vi "TCP-Main.vi"() -> ()   [LabVIEW 2014]
panel:
  out "读":string
  in  "Send":bool
  out "错误输出":errorcluster
  in  "错误输入（无错误）":errorcluster
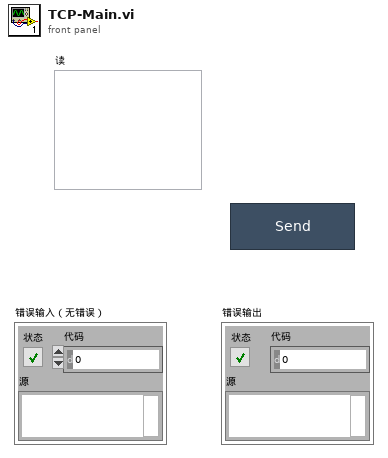
[diagram p1: front panel]
types:
  T1 = enum16{"Init", "Loop", "Write LOFF", "Write LON", "Read", "Exit", "Open", "Close"}
  T2 = enum16{"Standard", "Buffered", "CRLF", "Immediate"}
  T3 = enum32{"invalid app kind", "Development System", "Run Time System", "Student Edition", "Embedded LabVIEW", "Evaluation", "Custom"}
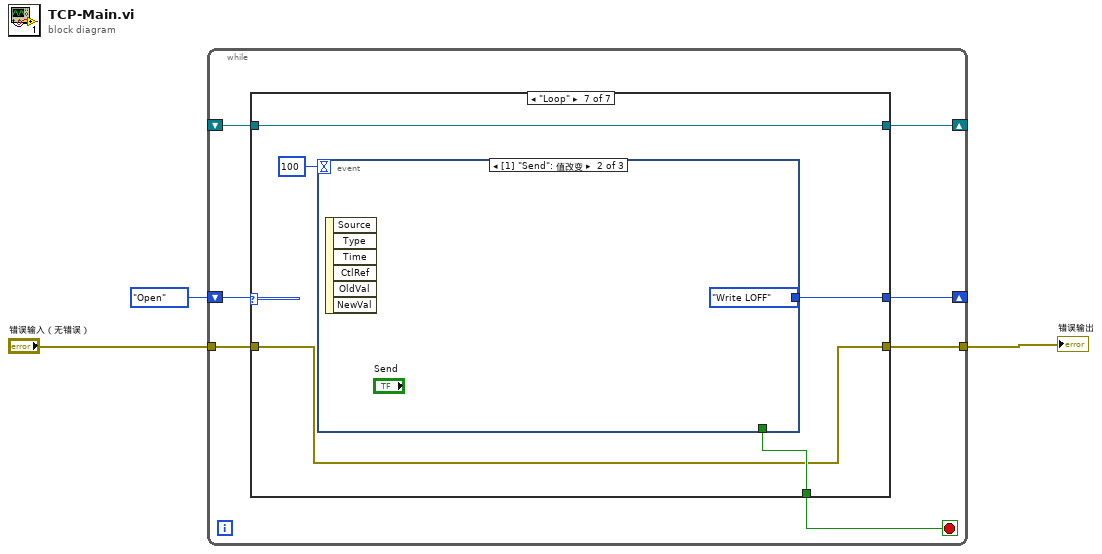
[diagram p0: block diagram]
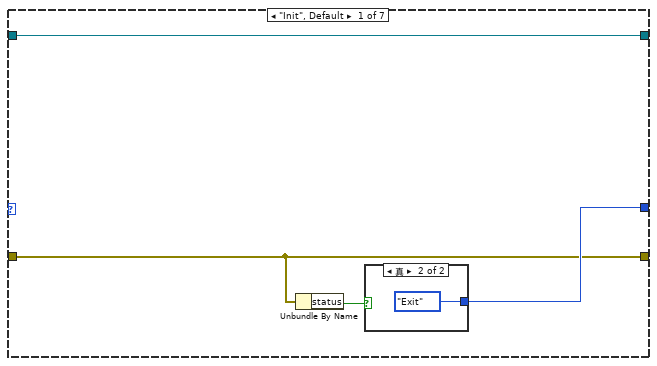
[diagram p2: hidden frame]
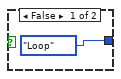
[diagram p3: hidden frame]
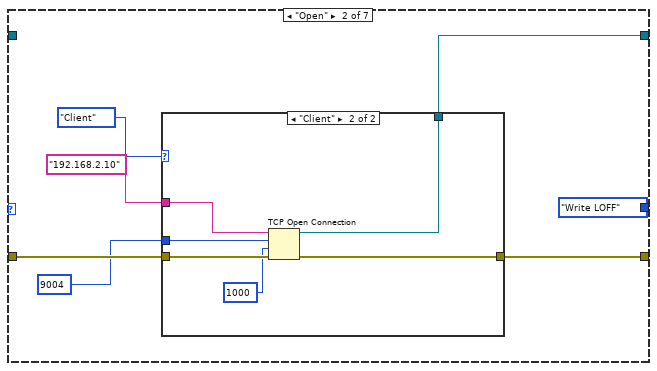
[diagram p4: hidden frame]
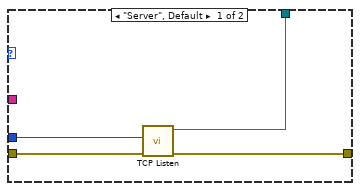
[diagram p5: hidden frame]
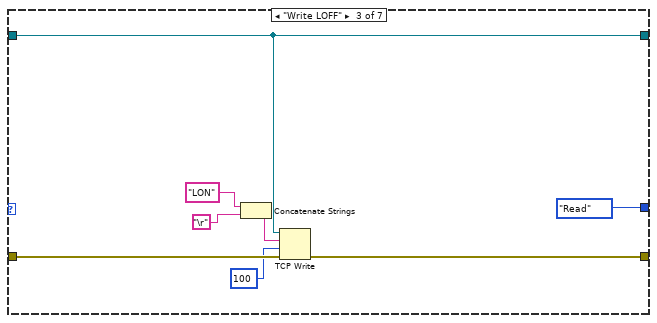
[diagram p6: hidden frame]
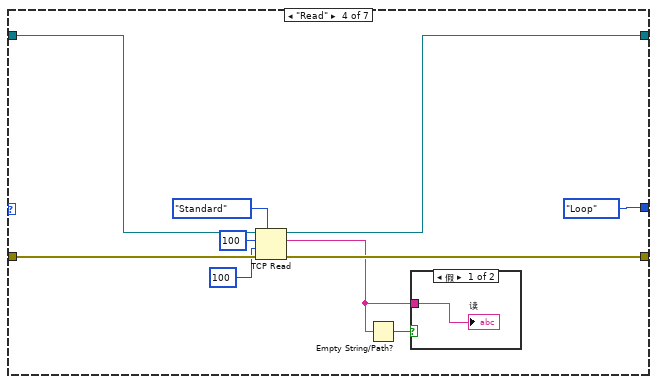
[diagram p7: hidden frame]
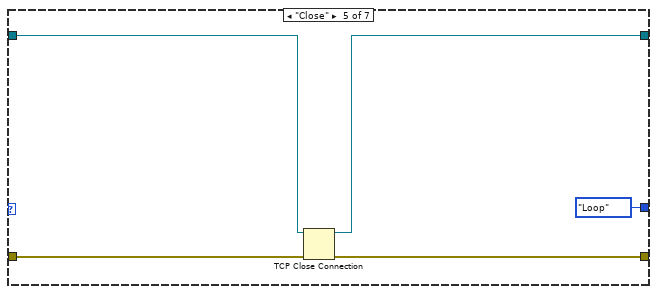
[diagram p9: hidden frame]
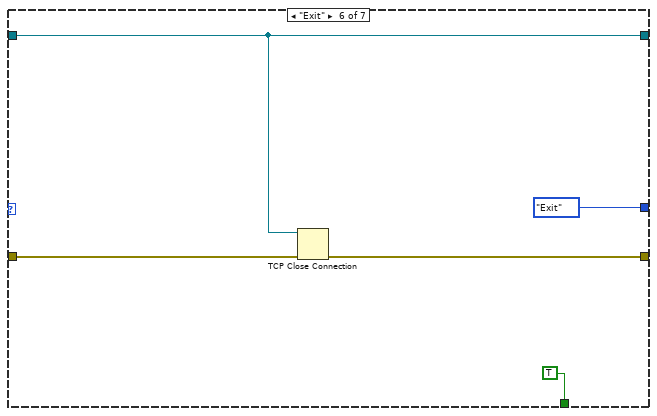
[diagram p10: hidden frame]
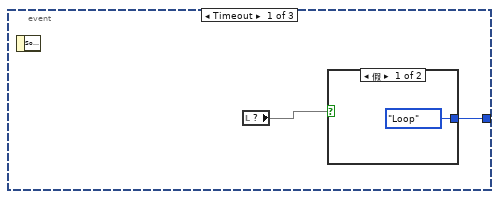
[diagram p11: hidden frame]
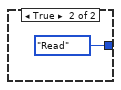
[diagram p12: hidden frame]
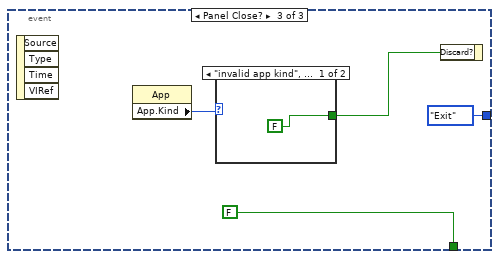
[diagram p13: hidden frame]
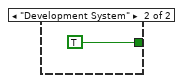
[diagram p14: hidden frame]
diagram:
  n1 = while {
    shift-right: [w9] -> _
    shift-left: T1."Open" -> [w10]
    shift-right: [w7] -> _
    shift-left: _ -> [w6]
    tunnel: "错误输入（无错误）" -> [w5]
    tunnel: [w4] -> w1
    stop <- w8 stop-if-true
    n2 = case shown="\"Loop\"" w10 {
      tunnel: [w13 T1."Write LOFF" T1."Read" T1."Loop" T1."Loop" T1."Exit" w65] -> w9
      tunnel: [_ _ _ _ _ TRUE w67] -> w8
      tunnel: [w11 w17 w40 w45 w53 w60 w64] -> w7
      tunnel: w6 -> [w11 _ w40 w42 w56 w60 w64]
      tunnel: w5 -> [w12 w21 w39 w49 w57 w59 w63]
      tunnel: [w12 w20 w38 w47 w55 w58 w63] -> w4
      frame "Init", Default {
        n3 = Unbundle By Name(w12) -> ("status"=w14:bool)
        n4 = case shown="真" w14 {
          tunnel: [T1."Loop" T1."Exit"] -> w13
          frame False {
          }
          frame True {
          }
        }
      }
      frame "Open" {
        n5 = case shown="\"Client\"" enum16{"Server", "Client"}."Client" ("类型") {
          tunnel: "192.168.2.10" ("IP") -> [_ w33]
          tunnel: w21 -> [w25 w32]
          tunnel: [w24 w31] -> w20
          tunnel: u16 9004 ("Port") -> [w27 w30]
          tunnel: [w26 w28] -> w17
          frame "Server", Default {
            n6 = call <vilib>:"TCP Listen.vi"("error in (no error)"=w25, "port"=w27) -> ("error out"=w24:errorcluster, "connection ID"=w26:refnum<k5>)  [unwired: 5 in, 3 out]
          }
          frame "Client" {
            n7 = TCP Open Connection(address=w33, remote port or service name=w30, timeout ms (60000)=1000 ("超时毫秒(60000)"), error in (no error)=w32) -> (connection ID=w28:refnum<k5>, error out=w31:errorcluster)  [unwired: 1 in]
          }
        }
      }
      frame "Write LOFF" {
        n8 = Concatenate Strings("LON" ("写"), "\r") -> (w36:string)
        n9 = TCP Write(connection ID=w40, data in=w36, error in (no error)=w39, 9:100 ("超时毫秒(25000)")) -> (error out=w38:errorcluster)  [unwired: 2 out]
      }
      frame "Read" {
        n10 = TCP Read(connection ID=w42, bytes to read=100 ("读取的字节"), error in (no error)=w49, 7:T2."Standard" ("模式（标准）"), 9:100 ("超时毫秒(25000)")) -> (connection ID out=w45:refnum<k5>, data out=w46:string, error out=w47:errorcluster)
        n11 = Empty String/Path?(string/path=w46) -> (empty?=w50:bool)
        n12 = case shown="假" w50 {
          tunnel: w46 -> [w52 _]
          frame False {
            "读" <- w52
          }
          frame True {
          }
        }
      }
      frame "Close" {
        n13 = TCP Close Connection(connection ID=w56, error in (no error)=w57) -> (connection ID out=w53:refnum<k5>, error out=w55:errorcluster)  [unwired: 1 in]
      }
      frame "Exit" {
        n14 = TCP Close Connection(connection ID=w60, error in (no error)=w59) -> (error out=w58:errorcluster)  [unwired: 1 in, 1 out]
      }
      frame "Loop" {
        n15 = event shown="[1] \"Send\": 值改变" {
          selector: _ -> [_ _ _]
          dyn-events: _ -> [_ _ _]
          timeout: 100 -> [_ _ _]
          tunnel: [_ _ FALSE] -> w67
          tunnel: [w69 T1."Write LOFF" T1."Exit"] -> w65
          event Timeout {
            n16 = event-data() -> ()  [unwired: 1 in, 1 out]
            n17 = local read item#-1() -> (w68)
            n18 = case shown="假" w68 {
              tunnel: [T1."Loop" T1."Read"] -> w69
              frame False {
              }
              frame True {
              }
            }
          }
          event "Send": Value Change {
            n19 = event-data() -> ()  [unwired: 1 in, 6 out]
          }
          event Panel Close? {
            n20 = event-data() -> ()  [unwired: 1 in, 4 out]
            n21 = property class="App"() -> ("App.Kind"=w75:T3)  [unwired: 2 in, 2 out]
            n22 = case shown="\"invalid app kind\", 默认" w75 {
              tunnel: [FALSE TRUE] -> w74
              frame "invalid app kind", Default {
              }
              frame "Development System" {
              }
            }
            n23 = event-data("Discard?"=w74) -> ()  [unwired: 1 in, 1 out]
          }
        }
      }
    }
  }
  "错误输出" <- w1
